vi "CommonVIs_GetModifierNames.vi"() -> (1 "ExatrModifiers":string[](array[string]), 2 "AllModifiers":string[](array[string]), 3 "AccessScopeModifiers":string[](array[string]))   [LabVIEW 2020]
uses:
  <resource>/Framework/Providers/Open_GDS/ClassProviders/Common/String/GDSString_AccessScopeModifierType.ctl
  <resource>/Framework/Providers/Open_GDS/ClassProviders/Common/String/GDSString_ModifierType.ctl
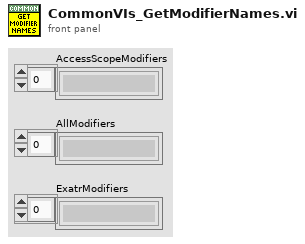
[diagram p1: front panel]
types:
  T1 = typedef "GDSString_ModifierType.ctl" = enum16{"abstract", "static", "final", "synchronized", "strictfp", "async", "const", "event", "extern", "new", "native ", "override", "partial", "readonly", "sealed", "unsafe", "virtual", "volatile"}
  T2 = typedef "GDSString_AccessScopeModifierType.ctl" = enum16{"public", "private", "protected", "internal"}
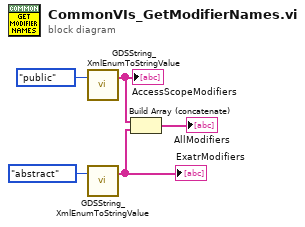
[diagram p0: block diagram]
diagram:
  n1 = call <resource>:"GDSString_XmlEnumToStringValue.vi"("EnumVariantIn(used if String is Empty)"=GDSString_AccessScopeModifierType."public" ("AccessScope")) -> ("EnumItems(string)"=w3:string[])  [unwired: 15 in, 3 out]
  "AccessScopeModifiers" <- w3
  n2 = call <resource>:"GDSString_XmlEnumToStringValue.vi"("EnumVariantIn(used if String is Empty)"=GDSString_ModifierType."abstract" ("Modifiers")) -> ("EnumItems(string)"=w4:string[])  [unwired: 15 in, 3 out]
  "ExatrModifiers" <- w4
  n3 = Build Array (concatenate)(w3, w4) -> (→"AllModifiers":string[])
